vi "eFGV -  AI Calibrated.vi"(6 "States":T1, 8 "Error In":errorcluster, 11 "AI Calibrated In":waveform(dbl)[](array[waveform])) -> (0 "Error Out":errorcluster, 2 "AI Calibrated Out":refnum<user-event>)   [LabVIEW 2020]
uses:
  Control/State - eFGV.ctl
  <vilib>/event_ctls.llb/usereventprio.ctl
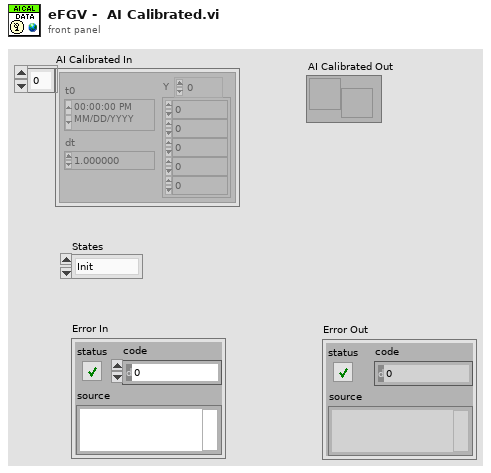
[diagram p1: front panel]
types:
  T1 = typedef "State - eFGV.ctl" = enum16{"Init", "Read", "Write", "Exit"}
  T2 = typedef "usereventprio.ctl" = enum32{"high priority", "normal priority"}
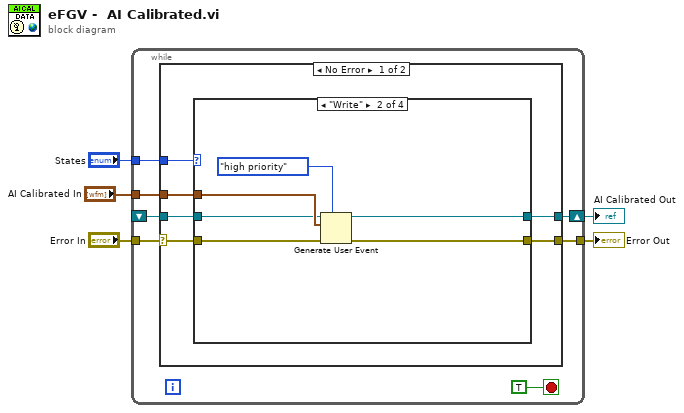
[diagram p0: block diagram]
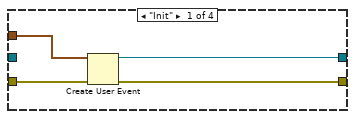
[diagram p2: hidden frame]
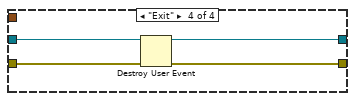
[diagram p4: hidden frame]
diagram:
  n1 = while {
    tunnel: "Error In" -> [w11]
    tunnel: [w10] -> w4
    tunnel: "States" -> [w9]
    tunnel: "AI Calibrated In" -> [w8]
    shift-right: [w7] -> w1
    shift-left: _ -> [w6]
    stop <- TRUE stop-if-true
    n2 = case shown="No Error" w11 {
      selector: w11 -> [w17 w35]
      tunnel: [w16 w35] -> w10
      tunnel: w9 -> [w18 _]
      tunnel: w8 -> [w15 _]
      tunnel: [w14 w34] -> w7
      tunnel: w6 -> [w13 w34]
      frame No Error {
        n3 = case shown="\"Write\"" w18 {
          tunnel: w17 -> [w22 w28 w30 w33]
          tunnel: [w21 w27 w30 w32] -> w16
          tunnel: w15 -> [w20 w26 _ _]
          tunnel: [w19 w24 w29 w31] -> w14
          tunnel: w13 -> [_ w25 w29 w31]
          frame "Init" {
            n4 = Create User Event(user event datatype=w20, error in=w22) -> (user event=w19:refnum<user-event>, error out=w21:errorcluster)
          }
          frame "Write" {
            n5 = Generate User Event(priority (normal)=usereventprio."high priority", user event=w25, event data cluster=w26, error in=w28) -> (user event out=w24:refnum<user-event>, error out=w27:errorcluster)
          }
          frame "Read", Default {
          }
          frame "Exit" {
            n6 = Destroy User Event(user event=w31, error in=w33) -> (error out=w32:errorcluster)
          }
        }
      }
      frame Error {
      }
    }
  }
  "Error Out" <- w4
  "AI Calibrated Out" <- w1
